vi "Create Data Channel Element.vi"(6 "Data Channel Parameters":T3, 7 "Settings":T1, 8 "Error In":errorcluster, 10 "Name":string, 11 "Refnum In":T8 format="%.0x") -> (0 "Error Out":errorcluster, 2 "Channel Refnum":T8 format="%.0x", 3 "Refnum Out":T8 format="%.0x")   [LabVIEW 2019, in "Instrument Addon Scripting API.lvlib"]
uses:
  Instrument Addon Scripting API.lvlib
  <vilib>/NI VeriStand/Custom Device API/Custom Device Item Ref.ctl
  Addon/Addon Shared/Types/Data Parameters.ctl
  Addon/Addon Shared/Types/Protocol Data Type.ctl
  Addon/Addon Shared/Types/Data Channel Type.ctl
  Addon/Addon Shared/Types/Type Cast Type.ctl
  Addon/Addon Shared/Types/Endian.ctl
  <vilib>/NI VeriStand/Custom Device API/Custom Device Channel.ctl
  <vilib>/NI VeriStand/Custom Device API/Custom Device Channel Type.ctl
  Addon/Addon Shared/Types/FG Control.ctl
  Addon/Addon Shared/SubVIs/Constants.vi
  <vilib>/NI VeriStand/Custom Device API/NI VeriStand - Get Item Property.vi
  <vilib>/NI VeriStand/Custom Device API/Get Item Property (U32).vi
  <vilib>/NI VeriStand/Custom Device API/Get Item Property (String).vi
  <vilib>/NI VeriStand/Custom Device API/Get Item Property (String Array).vi
  <vilib>/NI VeriStand/Custom Device API/NI VeriStand - Set Item Property.vi
  <vilib>/NI VeriStand/Custom Device API/Set Item Property (U32).vi
  <vilib>/NI VeriStand/Custom Device API/Set Item Property (String).vi
  <vilib>/NI VeriStand/Custom Device API/Set Item Property (String Array).vi
  Addon/Addon Shared/SubVIs/Set Channel Value Table.vi
  <vilib>/NI VeriStand/Custom Device API/NI VeriStand - Get Item Children.vi
  <vilib>/NI VeriStand/Custom Device API/NI VeriStand - Set Custom Device Channel Value Table.vi
  <vilib>/NI VeriStand/Custom Device API/Custom Device API.lvlib
  Addon/Addon Shared/Instrument Addon Shared.lvlib
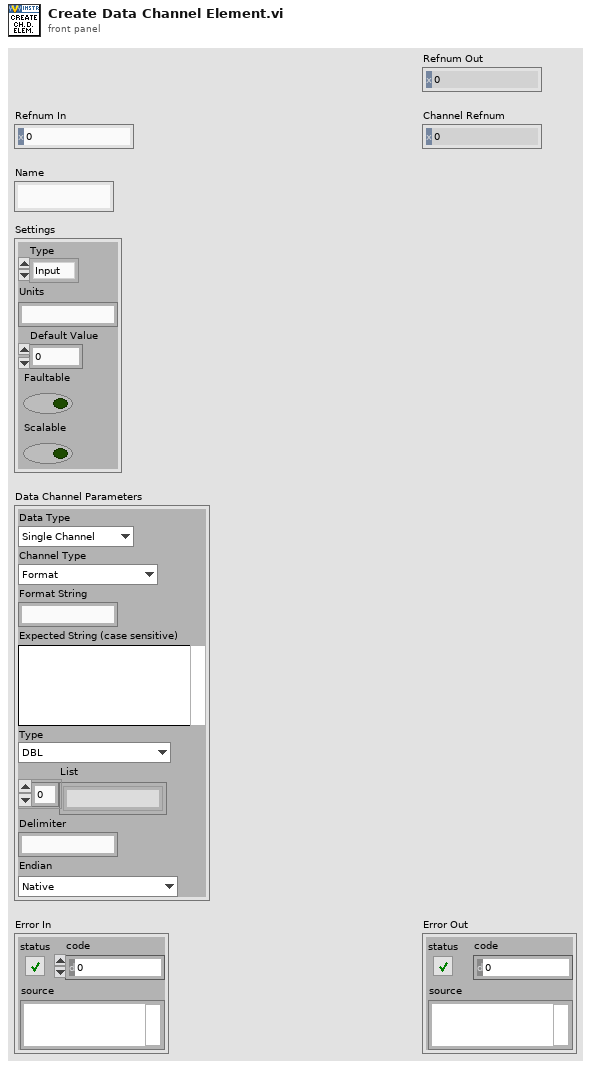
[diagram p1: front panel]
types:
  T1 = typedef "Custom Device API.lvlib/Custom Device Channel.ctl" = cluster{"Type":T2, "Units":string, "Default Value":dbl, "Faultable":bool, "Scalable":bool}
  T2 = typedef "Custom Device API.lvlib/Custom Device Channel Type.ctl" = enum16{"Input", "Output"}
  T3 = typedef "Instrument Addon Shared.lvlib/Data Parameters.ctl" = cluster{"Data Type":T4, "Channel Type":T5, "Format String":string, "Expected String":string, "Type":T6, "List":string[], "Delimiter":string, "Endian":T7}
  T4 = typedef "Instrument Addon Shared.lvlib/Protocol Data Type.ctl" = enum16{"Single Channel", "Array"}
  T5 = typedef "Instrument Addon Shared.lvlib/Data Channel Type.ctl" = enum16{"Format", "Comparison", "Type Cast", "Enumerated List"}
  T6 = typedef "Instrument Addon Shared.lvlib/Type Cast Type.ctl" = enum16{"DBL", "SGL", "U64", "U32", "U16", "U8", "I64", "I32", "I16", "I8"}
  T7 = typedef "Instrument Addon Shared.lvlib/Endian.ctl" = enum16{"Native", "Little", "Big"}
  T8 = typedef "Custom Device API.lvlib/Custom Device Item Ref.ctl" = u64
  T9 = typedef "Instrument Addon Shared.lvlib/FG Control.ctl" = enum16{"Get", "Set"}
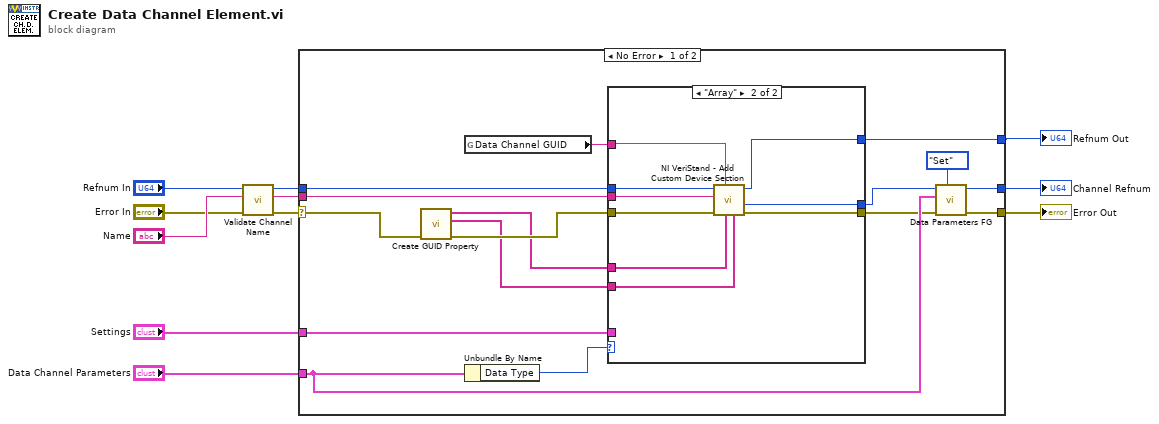
[diagram p0: block diagram]
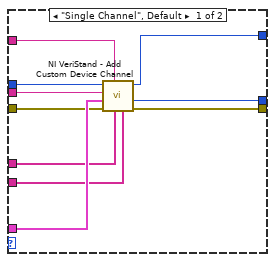
[diagram p2: hidden frame]
diagram:
  n1 = call "Validate Channel Name.vi"("error in (no error)"="Error In", "Name In"="Name", "Refnum In"="Refnum In") -> ("error out"=w3:errorcluster, "Name Out"=w4:string, "Refnum Out"=w5:T8)  [unwired: 6 in]
  n2 = case shown="No Error" w3 {
    selector: w3 -> [w17 w48]
    tunnel: [w20 _] -> w11
    tunnel: "Settings" -> [w27 _]
    tunnel: [w21 w48] -> w9
    tunnel: "Data Channel Parameters" -> [w24 _]
    tunnel: w5 -> [w15 w47]
    tunnel: w4 -> [w16 _]
    tunnel: [w22 w47] -> w7
    frame No Error {
      n3 = call "Create GUID Property.vi"("error in (no error)"=w17) -> ("error out"=w14:errorcluster, "property values"=w12:string[], "property names"=w13:string[])  [unwired: 8 in]
      n4 = global read "Constants.vi" "Data Channel GUID"() -> (w23:string)
      n5 = Unbundle By Name(w24) -> ("Data Type"=w25:T4)
      n6 = case shown="\"Array\"" w25 {
        tunnel: w16 -> [w37 w46]
        tunnel: w27 -> [w36 _]
        tunnel: [w35 w41] -> w18
        tunnel: [w34 w42] -> w19
        tunnel: w14 -> [w33 w44]
        tunnel: w15 -> [w32 w43]
        tunnel: w23 -> [w31 w45]
        tunnel: [w30 w40] -> w22
        tunnel: w13 -> [w29 w39]
        tunnel: w12 -> [w28 w38]
        frame "Single Channel", Default {
          n7 = call <vilib>:"NI VeriStand - Add Custom Device Channel.vi"("Property Values"=w28, "Property names"=w29, "GUID (Default Channel)"=w31, "error in (no error)"=w33, "Channel"=w36, "Channel Name"=w37, "Parent Ref in"=w32) -> ("error out"=w34:errorcluster, "Channel Ref"=w35:T8, "Parent Ref out"=w30:T8)  [unwired: 1 in, 1 out]
        }
        frame "Array" {
          n8 = call <vilib>:"NI VeriStand - Add Custom Device Section.vi"("Property Values"=w38, "Property names"=w39, "GUID (Default Section)"=w45, "error in (no error)"=w44, "Section Name"=w46, "Parent Ref in"=w43) -> ("error out"=w42:errorcluster, "Section Ptr"=w41:T8, "Parent Ref out"=w40:T8)  [unwired: 2 in, 1 out]
        }
      }
      n9 = call "Data Parameters FG.vi"("Action"=FG_Control."Set", "error in (no error)"=w19, "Data Parameters"=w24, "Item Ref in"=w18) -> ("error out"=w21:errorcluster, "Item Ref out"=w20:T8)  [unwired: 5 in, 1 out]
    }
    frame Error {
    }
  }
  "Channel Refnum" <- w11
  "Refnum Out" <- w7
  "Error Out" <- w9
